vi "DPCal-Config.vi"(0 "Speakers":string[](array[string]), 1 "freqs":dbl[](array[numeric]), 2 "Attenuation (dB)":dbl[](array[numeric]), 5 "Mic":string, 7 "Sampling Rate (Hz)":dbl=200000.0, 9 "Npts":i32=10000, 11 "error in (no error)":errorcluster, 12 "Nbuf":i32=10000) -> (8 "Signal out":dbl[][](array[numeric]), 15 "error out":errorcluster)   [LabVIEW 2020]
uses:
  epl-vi-lib/Signal Synthesis VIs/4th Generation/Classes/Gate/Gate.lvclass/Gate.ctl
  bc6414e4-3673-4db9-9987-8075f6ebf4c6.vi
  fabe2aeb-84af-45f9-a318-4647dc3326b9.vi
  epl-vi-lib/Signal Synthesis VIs/4th Generation/Common/CommonSig-Apply Ramp (2D).vi
  50cf06c4-ddb6-403d-aefe-4311d7d37b60.vi
  8a331112-bbc1-4753-9b51-6dceaaeb95e8.vi
  epl-vi-lib/Signal Synthesis VIs/4th Generation/Common/CommonSig-Apply Ramp (2D).vi/00fa021d-ebe0-42e5-9c35-5538040c7da1.vi
  epl-vi-lib/Signal Synthesis VIs/4th Generation/Classes/Gate/Write Ramp (ms).vi
  epl-vi-lib/Signal Synthesis VIs/4th Generation/Classes/Gate/Write Down (ms).vi
  epl-vi-lib/Signal Synthesis VIs/4th Generation/Classes/Gate/Write Asymmetric.vi
  epl-vi-lib/Signal Synthesis VIs/4th Generation/Classes/Gate/Write Shape.vi
  epl-vi-lib/Signal Synthesis VIs/4th Generation/Classes/Gate/Write Duration (ms).vi
  epl-vi-lib/PXI DAQ VIs/AIDI/AIDI-Engine.vi
  epl-vi-lib/Signal Synthesis VIs/4th Generation/Classes/Gate/Create.vi
  epl-vi-lib/Signal Synthesis VIs/4th Generation/Classes/Gate/Apply.vi
  epl-vi-lib/PXI DAQ VIs/AODO/AODO-Engine.vi
  <vilib>/Analysis/NI_AALBase.lvlib
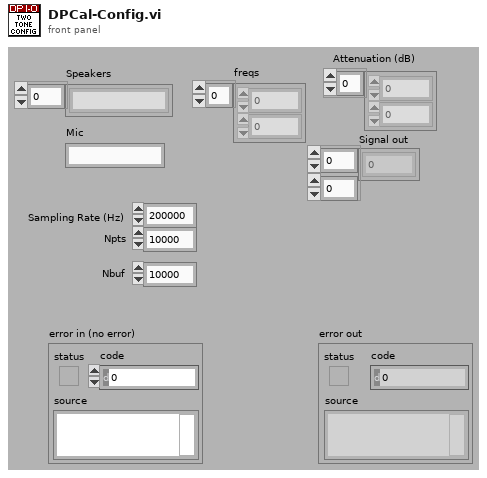
[diagram p1: front panel]
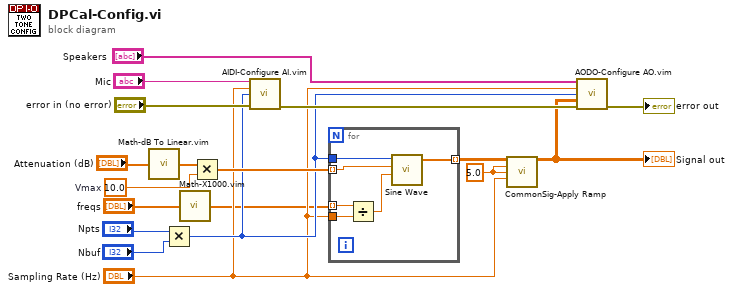
[diagram p0: block diagram]
diagram:
  w3 = 5.0 ("Ramp up (ms)")
  w9 = 10.0  # Vmax
  n1 = call "Math-dB To Linear.vim"("dB"="Attenuation (dB)") -> ("linear"=w10:dbl[])
  n2 = Multiply(x="Npts", y="Nbuf") -> (x*y=w6:i32)
  n3 = call "Math-X1000.vim"("X"="freqs") -> ("1000X"=w1:dbl[])
  n4 = Multiply(x=w10, y=w9) -> (x*y=w7:dbl[])
  n5 = call "AIDI-Configure AI.vim"("AI.Channels"="Mic", "AI.Fs (Hz)"="Sampling Rate (Hz)", "AI.Npts"=w6, "error in (no error)"="error in (no error)") -> ("error out"=w13:errorcluster)  [unwired: 11 in]
  n6 = for {
    tunnel: w1 -> [w22] mode=indexing
    tunnel: w7 -> [w23] mode=indexing
    tunnel: w6 -> [w24]
    tunnel: "Sampling Rate (Hz)" -> [w20]
    tunnel: [w19] -> w5 mode=indexing
    n7 = Divide(x=w22, y=w20) -> (x/y=w21:dbl)
    n8 = call <vilib>:"Sine Wave.vi"("samples"=w24, "amplitude"=w23, "frequency"=w21) -> ("sine wave"=w19:dbl[])  [unwired: 2 in, 2 out]
  }
  n9 = call-poly "CommonSig-Apply Ramp.vi"("Array in"=w5, "Ramp up (ms)"=w3, "Ramp down (ms)"=w3, "Fs (Hz)"="Sampling Rate (Hz)") -> ("Array out"=w4:dbl[][])  [unwired: 10 in, 1 out]
  "Signal out" <- w4
  n10 = call "AODO-Configure AO.vim"("AO.Channels"="Speakers", "AO.Fs (Hz)"="Sampling Rate (Hz)", "AO.Npts"=w6, "AO"=w4, "error in (no error)"=w13) -> ("error out"=→"error out":errorcluster)  [unwired: 10 in]
